vi "test Parse Capabilities Files.vi"(8 "error in (no error)":errorcluster, 11 "TestCase in":refnum<class "SLSC EDS Unit Tests.lvclass">) -> (0 "error out":errorcluster, 3 "TestCase out":refnum<class "SLSC EDS Unit Tests.lvclass">)   [LabVIEW 2015, in "SLSC EDS Unit Tests.lvclass"]
uses:
  SLSC EDS Unit Tests.lvclass
  SLSC EDS API/JSON parsing/EDSjsonStructure.ctl
  SLSC EDS API/JSON parsing/enum.ctl
  SLSC EDS API/JSON parsing/property.ctl
  SLSC EDS API/JSON parsing/command.ctl
  SLSC EDS API/JSON parsing/scale.ctl
  SLSC EDS API/JSON parsing/physicalChannel.ctl
  SLSC EDS API/JSON parsing/register.ctl
  <vilib>/addons/_JKI Toolkits/VI Tester/TestCase.llb/TestCase.lvclass
panel:
  out "Pass?":bool
  out "Array 2":errorcluster[](array[cluster])
  out "appended array":path[](array[path])
  out "Array":T1[](array[typedef])
  # "not working\nregisterMap->registers->initialValue"
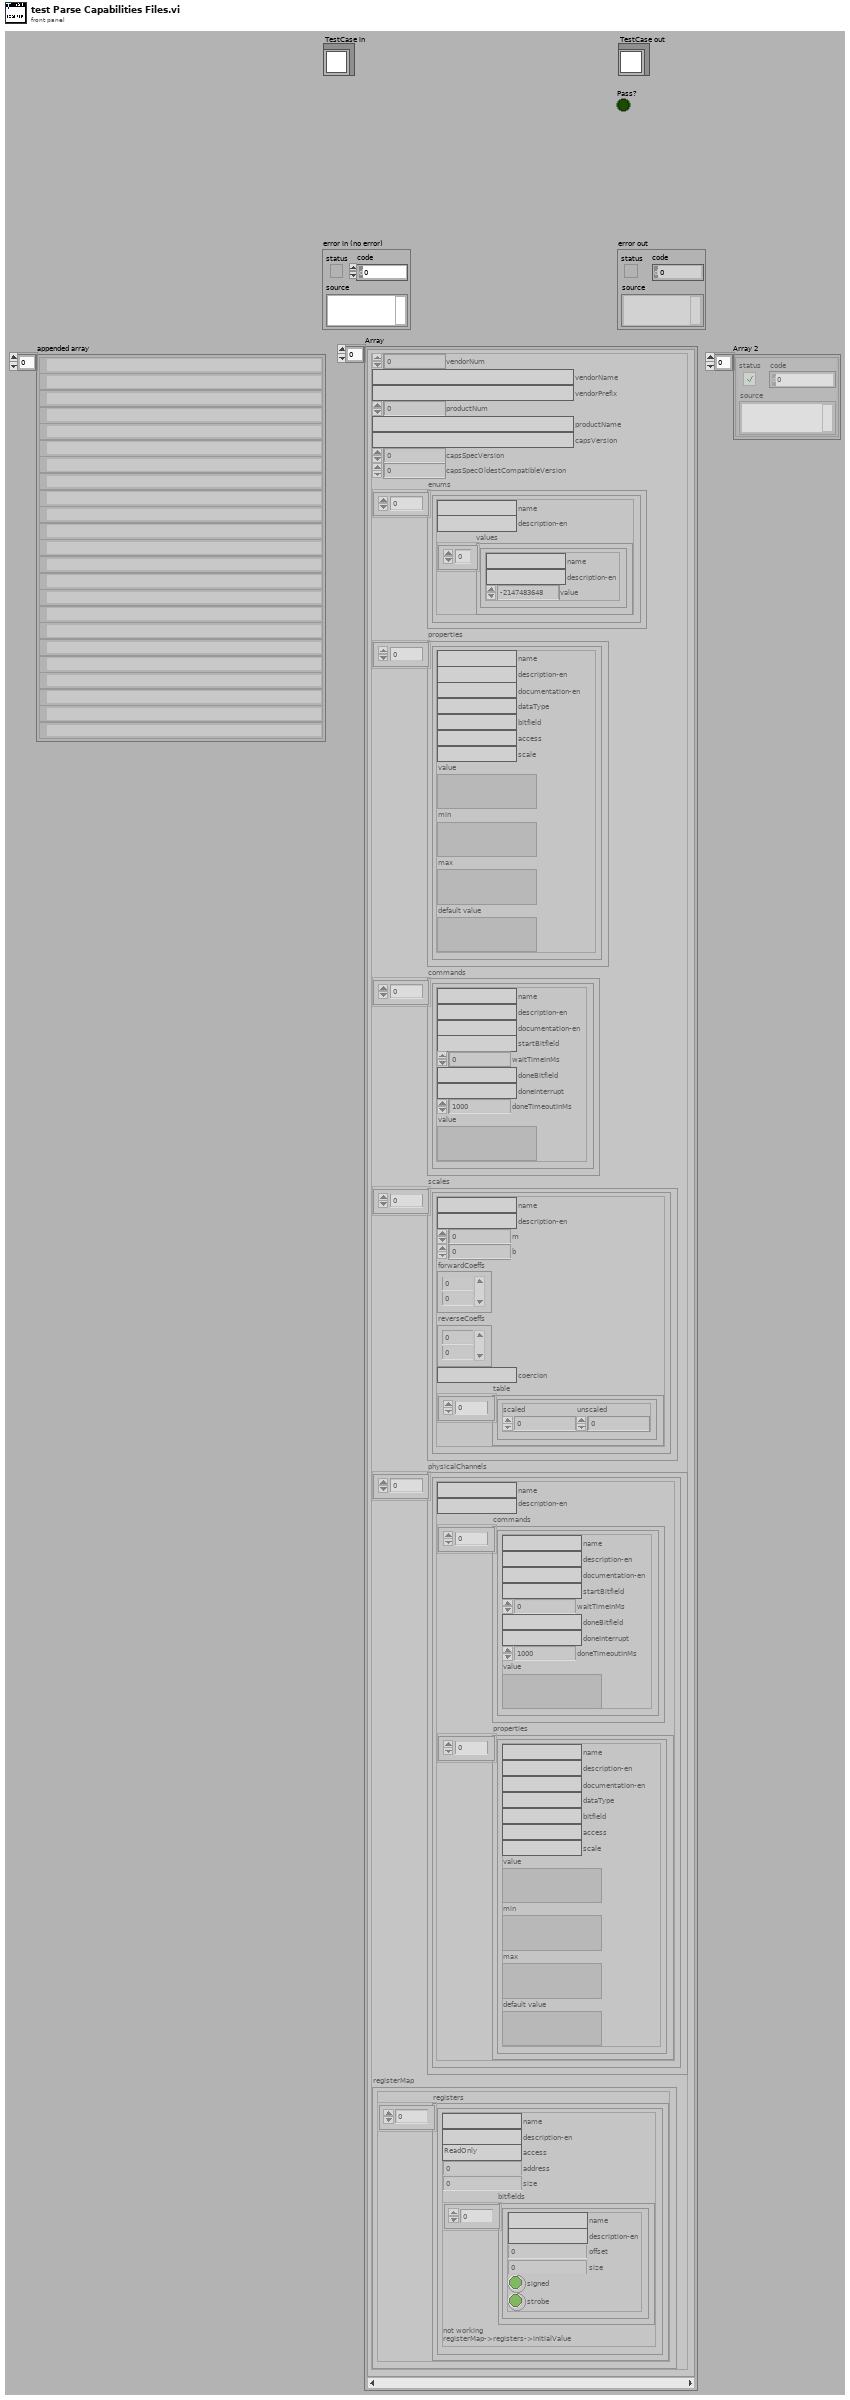
[diagram p1: front panel]
types:
  T1 = typedef "EDSjsonStructure.ctl" = cluster{"vendorNum":u32, "vendorName":string, "vendorPrefix":string, "productNum":u32, "productName":string, "capsVersion":string, "capsSpecVersion":u32, "capsSpecOldestCompatibleVersion":u32, "enums":T2[], "properties":T3[], "commands":T4[], "scales":T5[], "physicalChannels":T6[], "registerMap":cluster{"registers":T7[]}}
  T2 = typedef "enum.ctl" = cluster{"name":string, "description-en":string, "values":cluster{"name":string, "description-en":string, "value":i32}[]}
  T3 = typedef "property.ctl" = cluster{"name":string, "description-en":string, "documentation-en":string, "dataType":string, "bitfield":string, "access":string, "scale":string, "value":variant, "min":variant, "max":variant, "default value":variant}
  T4 = typedef "command.ctl" = cluster{"name":string, "description-en":string, "documentation-en":string, "startBitfield":string, "waitTimeInMs":i32, "doneBitfield":string, "doneInterrupt":string, "doneTimeoutInMs":i32, "value":variant}
  T5 = typedef "scale.ctl" = cluster{"name":string, "description-en":string, "m":dbl, "b":dbl, "forwardCoeffs":dbl[], "reverseCoeffs":dbl[], "coercion":string, "table":cluster{"scaled":dbl, "unscaled":dbl}[]}
  T6 = typedef "physicalChannel.ctl" = cluster{"name":string, "description-en":string, "commands":T4[], "properties":T3[]}
  T7 = typedef "register.ctl" = cluster{"name":string, "description-en":string, "access":string, "address":u32, "size":u32, "bitfields":cluster{"name":string, "description-en":string, "offset":u32, "size":u32, "signed":bool, "strobe":bool}[]}
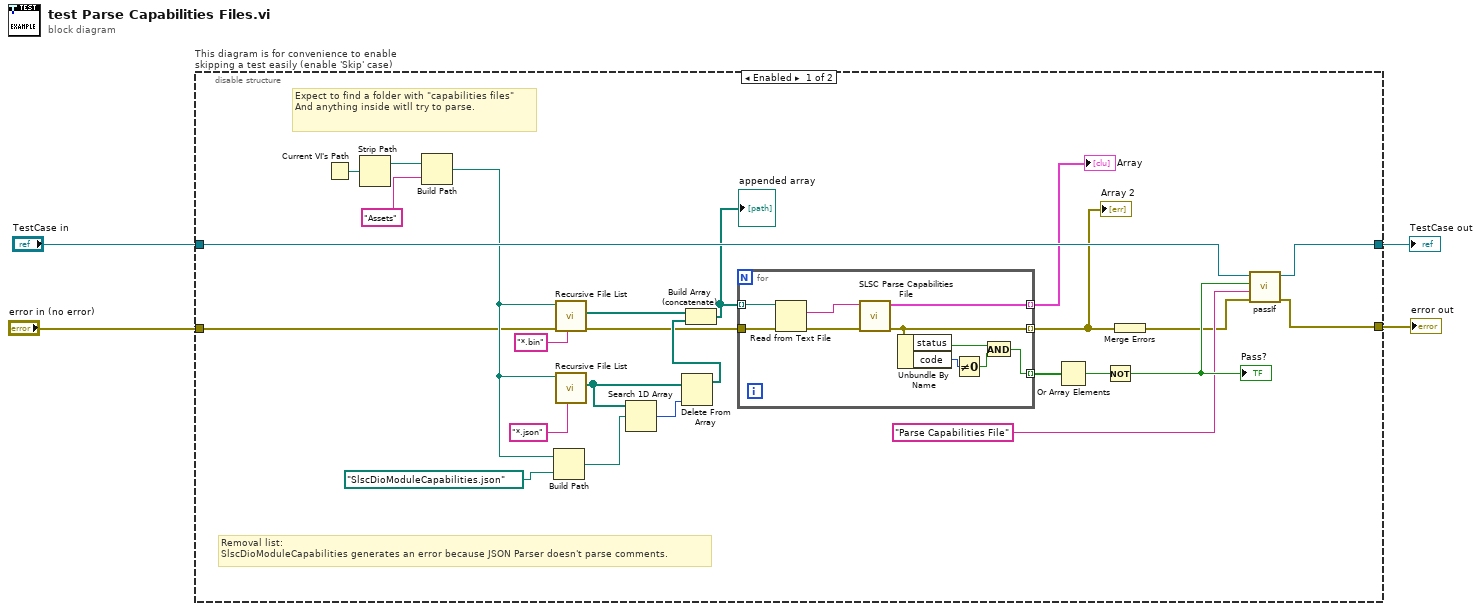
[diagram p0: block diagram]
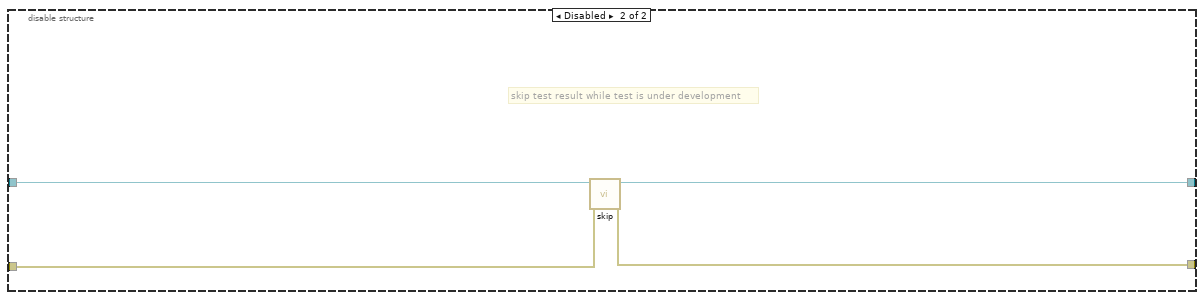
[diagram p2: hidden frame]
diagram:
  n1 = disable-structure "This diagram is for convenience to enable skipping a test easily (enable 'Skip' case)" shown="Enabled" {
    disable-tunnel: "TestCase in" -> [w29 w43]
    disable-tunnel: [w28 w41] -> w1
    disable-tunnel: [w27 w42] -> w3
    disable-tunnel: "error in (no error)" -> [w10 w40]
    frame Enabled {
      # "Expect to find a folder with \"capabilities files\" \nAnd anything inside witll try to parse."
      # "Removal list:\nSlscDioModuleCapabilities generates an error because JSON Parser doesn't parse comments."
      n2 = Current VI's Path() -> (path=w26:path)
      n3 = Strip Path(path=w26) -> (stripped path=w15:path)  [unwired: 1 out]
      n4 = Build Path(base path=w15, name or relative path="Assets") -> (appended path=w12:path)
      n5 = Build Path(base path=w12, name or relative path=path "SlscDioModuleCapabilities.json" ("element")) -> (appended path=w11:path)
      n6 = call <vilib>:"Recursive File List.vi"("pattern"="*.bin", "error in (no error)"=w10, "Folder Path"=w12) -> ("error out"=w7:errorcluster, "All Files in Dir"=w24:path[])  [unwired: 4 in, 3 out]
      n7 = call <vilib>:"Recursive File List.vi"("pattern"="*.json", "Folder Path"=w12) -> ("All Files in Dir"=w18:path[])  [unwired: 5 in, 4 out]
      n8 = Search 1D Array(1D array=w18, element=w11) -> (index of element=w20:i32)  [unwired: 1 in]
      n9 = Delete From Array(array=w18, index=w20) -> (array with subset deleted=w16:path[])  [unwired: 1 in, 1 out]
      n10 = Build Array (concatenate)(w24, w16) -> (w22:path[])
      "appended array" <- w22
      n11 = for {
        tunnel: w22 -> [w39] mode=indexing
        tunnel: [w37] -> w23 mode=indexing
        tunnel: [w32] -> w19 mode=indexing
        tunnel: [w31] -> w6 mode=indexing
        tunnel: w7 -> [w30]
        n12 = Read from Text File(file (use dialog)=w39, error in=w30) -> (text=w38:string, error out=w36:errorcluster)  [unwired: 2 in, 2 out]
        n13 = call "SLSC Parse Capabilities File.vi"("error in"=w36, "module capabilities JSON string"=w38) -> ("error out"=w31:errorcluster, "SLSC EDS module"=w37:T1)  [unwired: 8 in]
        n14 = Unbundle By Name(w31) -> ("status"=w35:bool, "code"=w34:i32)
        n15 = Not Equal To 0?(x=w34) -> (x != 0?=w33:bool)
        n16 = And(x=w35, y=w33) -> (x .and. y?=w32:bool)
      }
      "Array" <- w23
      "Array 2" <- w6
      n17 = Or Array Elements(Boolean array=w19) -> (logical OR=w17:bool)
      n18 = Not(x=w17) -> (.not. x?=w9:bool)
      "Pass?" <- w9
      n19 = Merge Errors(w6) -> (w5:errorcluster)
      n20 = call-dynamic "passIf.vi"("error in (no error)"=w5, "message (\"\")"="Parse Capabilities File" ("message (\"\")"), "pass"=w9, "TestCase in"=w29) -> ("error out"=w27:errorcluster, "TestCase out"=w28:refnum<class "SLSC EDS Unit Tests.lvclass">)  [unwired: 6 in]
    }
    frame Disabled {
      # "skip test result while test is under development"
      n21 = call <vilib>:"skip.vi"("error in (no error)"=w40, "TestCase in"=w43) -> ("error out"=w42:errorcluster, "TestCase out"=w41:refnum<class "SLSC EDS Unit Tests.lvclass">)  [unwired: 8 in]
    }
  }
  "error out" <- w3
  "TestCase out" <- w1
